vi "sub build c data.vi"(8 "error in":errorcluster, 11 "<c> data":T1) -> (0 "error out":errorcluster, 3 "<c> string":string)   [LabVIEW 2018, in "Frame Analizer.lvclass"]
uses:
  Frame Analizer.lvclass
  frame c data.ctl
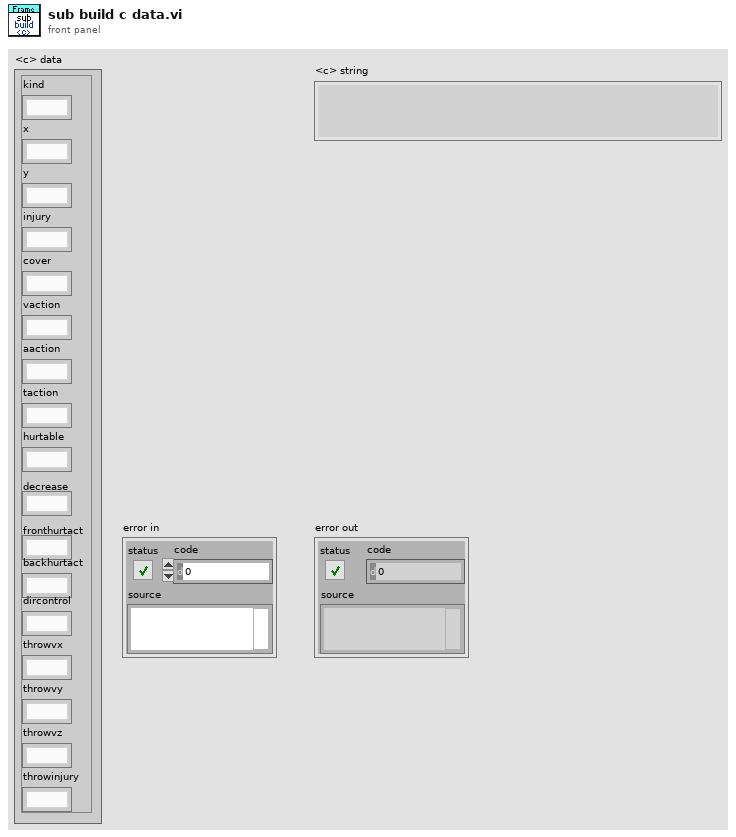
[diagram p1: front panel]
types:
  T1 = typedef "Frame Analizer.lvclass/frame c data.ctl" = cluster{"kind":string, "x":string, "y":string, "injury":string, "cover":string, "vaction":string, "aaction":string, "taction":string, "hurtable":string, "decrease":string, "fronthurtact":string, "backhurtact":string, "dircontrol":string, "throwvx":string, "throwvy":string, "throwvz":string, "throwinjury":string}
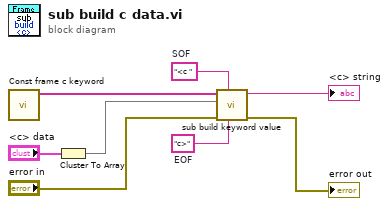
[diagram p0: block diagram]
diagram:
  w3 = "c>"  # EOF
  w4 = "<c "  # SOF
  n1 = call "Const frame c keyword.vi"() -> ("Const frame c keyword"=w1:string[])  [unwired: 11 in]
  n2 = Cluster To Array(cluster="<c> data") -> (array=w7:string[])
  n3 = call "sub build keyword value.vi"("EOF"=w3, "SOF"=w4, "error in"="error in", "value"=w7, "keyword"=w1) -> ("error out"=→"error out":errorcluster, "keyword value string"=→"<c> string":string)  [unwired: 5 in]
